vi "Module ID.vi"(11 "PluginGUI in":refnum<class "PluginGUI.lvclass">) -> (2 "Module ID":string)   [LabVIEW 2020, in "VolatusGUI.lvlib" / "PluginGUI.lvclass"]
uses:
  PluginGUI.lvclass
  C:/dev/lv20CE/relink/lv-volatus/Volatus/Module/Module.lvclass
  PluginGUI.lvclass/PluginGUI.ctl
  Volatus/Module/Module.lvclass/Module.ctl
  VolatusConfig/VolatusConfigElement/VolatusConfigElement.lvclass/VolatusConfigElement.ctl
  Volatus/Module/Config.vi
  VolatusConfig/VolatusConfigElement/Element.vi
  VolatusConfig/Task/Task Config.lvclass
  C:/dev/lv20CE/relink/lv-volatus/VolatusConfig/VolatusConfigElement/VolatusConfigElement.lvclass
  Volatus/Module/Module.lvclass
  VolatusConfig/VolatusConfigElement/VolatusConfigElement.lvclass
  C:/dev/lv20CE/relink/lv-volatus/VolatusGUI/PluginGUI/PluginGUI.lvclass
  C:/dev/lv20CE/relink/lv-volatus/VolatusConfig/Task/Task Config.lvclass
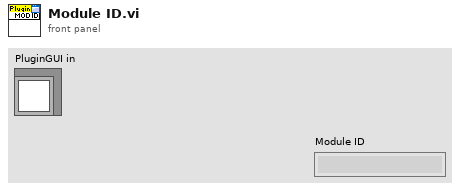
[diagram p1: front panel]
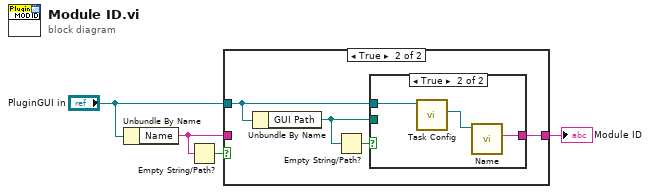
[diagram p0: block diagram]
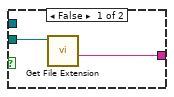
[diagram p3: hidden frame]
diagram:
  n1 = Unbundle By Name("PluginGUI in") -> ("Name"=w1:string)
  n2 = Empty String/Path?(string/path=w1) -> (empty?=w2:bool)
  n3 = case shown="True" w2 {
    tunnel: [w5 w7] -> w4
    tunnel: "PluginGUI in" -> [_ w6]
    tunnel: w1 -> [w5 _]
    frame False {
    }
    frame True {
      n4 = Unbundle By Name(w6) -> ("GUI Path"=w8:path)
      n5 = Empty String/Path?(string/path=w8) -> (empty?=w9:bool)
      n6 = case shown="True" w9 {
        tunnel: w8 -> [w11 _]
        tunnel: [w10 w13] -> w7
        tunnel: w6 -> [_ w12]
        frame False {
          n7 = call <vilib>:"Get File Extension.vi"("file"=w11) -> ("filename without extension"=w10:string)  [unwired: 6 in, 4 out]
        }
        frame True {
          n8 = call "Task Config.vi"("Module in"=w12) -> ("Task Config"=w14:refnum<class "Task Config.lvclass">)  [unwired: 8 in, 2 out]
          n9 = call "Name.vi"("VolatusConfigElement in"=w14) -> ("Name"=w13:string)  [unwired: 8 in, 2 out]
        }
      }
    }
  }
  "Module ID" <- w4
